vi "Sync Parent Symbols.vi"(8 "error in":errorcluster, 10 "Child Tag_LVOOP":refnum<class "Tree Tag Class.lvclass">, 11 "Tree_LVOOP in":refnum<class "Tree Class.lvclass">) -> (0 "error out":errorcluster, 3 "Tree_LVOOP out":refnum<class "Tree Class.lvclass">)   [LabVIEW 2012, in "Tree Tools.lvlib" / "Tree Class.lvclass"]
uses:
  Tree Class.lvclass
  Tree Tag Class/Tree Tag Class.lvclass
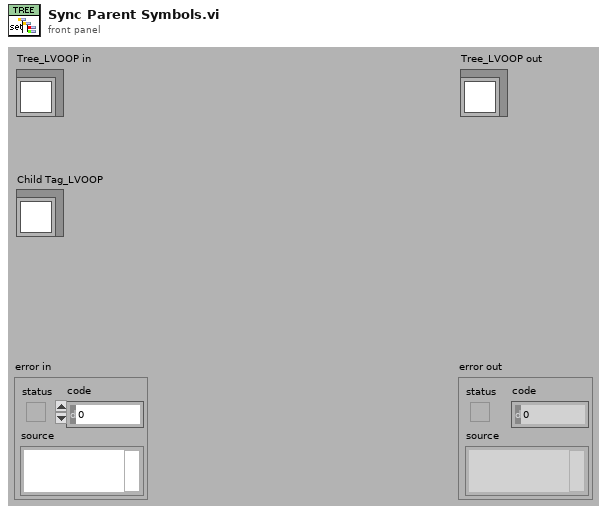
[diagram p1: front panel]
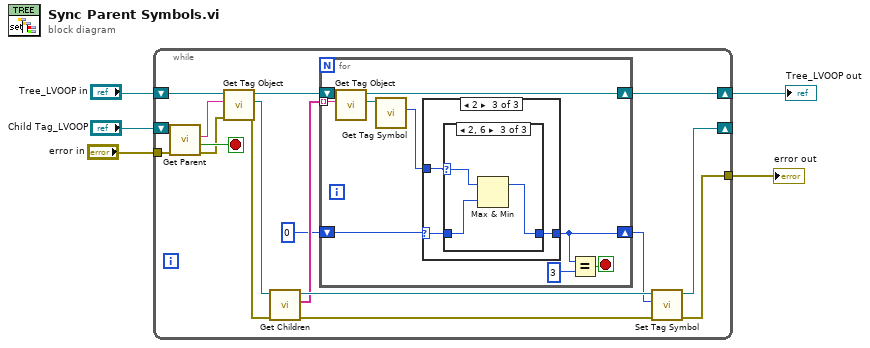
[diagram p0: block diagram]
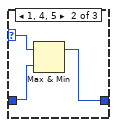
[diagram p6: hidden frame]
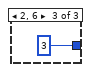
[diagram p7: hidden frame]
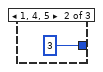
[diagram p9: hidden frame]
diagram:
  n1 = while {
    shift-right: [w18] -> _
    shift-left: "Child Tag_LVOOP" -> [w22]
    tunnel: "error in" -> [w11]
    tunnel: [w7] -> w1
    shift-right: [w6] -> w3
    shift-left: "Tree_LVOOP in" -> [w20]
    stop <- w21 stop-if-true
    n2 = call-dynamic "Get Parent.vi"("error in (no error)"=w11, "Tag_LVOOP in"=w22) -> ("error out"=w10:errorcluster, "Topmost?"=w21:bool, "Parent Tag string"=w19:string)  [unwired: 6 in, 1 out]
    n3 = call-dynamic "Get Tag Object.vi"("error in (no error)"=w10, "Tag (string)"=w19, "Tree_LVOOP in"=w20) -> ("error out"=w9:errorcluster, "Tag"=w17:refnum<class "Tree Tag Class.lvclass">, "Tree_LVOOP out"=w15:refnum<class "Tree Class.lvclass">)  [unwired: 1 in, 5 out]
    n4 = call-dynamic "Get Children.vi"("error in (no error)"=w9, "Tag_LVOOP in"=w17) -> ("error out"=w8:errorcluster, "Children Tag Strings"=w14:string[], "Tag_LVOOP out"=w16:refnum<class "Tree Tag Class.lvclass">)  [unwired: 6 in, 1 out]
    n5 = for {
      tunnel: w14 -> [w30] mode=indexing
      shift-right: [w24] -> w12
      shift-left: 0 ("y") -> [w26]
      shift-right: [w23] -> w6
      shift-left: w15 -> [w31]
      stop <- w28 stop-if-true
      n6 = call-dynamic "Get Tag Object.vi"("Tag (string)"=w30, "Tree_LVOOP in"=w31) -> ("Tag"=w29:refnum<class "Tree Tag Class.lvclass">, "Tree_LVOOP out"=w23:refnum<class "Tree Class.lvclass">)  [unwired: 2 in, 6 out]
      n7 = call-dynamic "Get Tag Symbol.vi"("Tag_LVOOP in"=w29) -> ("Symbol Index"=w25:i32)  [unwired: 8 in, 2 out]
      n8 = case shown="2" w26 {
        selector: w26 -> [w33 w39 w47]
        tunnel: w25 -> [w34 w40 w48]
        tunnel: [w32 w38 w46] -> w24
        frame 0, Default {
          n9 = case shown="默认" w34 {
            selector: w34 -> [_ w36 w37]
            tunnel: w33 -> [w35 _ _]
            tunnel: [w35 w36 w37] -> w32
            frame Default {
            }
            frame 1, 4, 5 {
            }
            frame 2, 6 {
            }
          }
        }
        frame 1 {
          n10 = case shown="默认" w40 {
            selector: w40 -> [_ w44 _]
            tunnel: w39 -> [w41 w43 _]
            tunnel: [w41 w42 3 ("y")] -> w38
            frame Default {
            }
            frame 1, 4, 5 {
              n11 = Max & Min(x=w44, y=w43) -> (max(x,y)=w42:i32)  [unwired: 1 out]
            }
            frame 2, 6 {
            }
          }
        }
        frame 2 {
          n12 = case shown="2, 6" w48 {
            selector: w48 -> [_ _ w53]
            tunnel: w47 -> [w49 _ w52]
            tunnel: [w49 3 ("y") w51] -> w46
            frame Default {
            }
            frame 1, 4, 5 {
            }
            frame 2, 6 {
              n13 = Max & Min(x=w53, y=w52) -> (max(x,y)=w51:i32)  [unwired: 1 out]
            }
          }
        }
      }
      n14 = Equal?(x=w24, y=3) -> (x = y?=w28:bool)
    }
    n15 = call-dynamic "Set Tag Symbol.vi"("error in (no error)"=w8, "Symbol Index"=w12, "Tag_LVOOP in"=w16) -> ("error out"=w7:errorcluster, "Tag_LVOOP out"=w18:refnum<class "Tree Tag Class.lvclass">)  [unwired: 7 in]
  }
  "error out" <- w1
  "Tree_LVOOP out" <- w3
